vi "Multicolumn Sort.vi"(10 "Imported Details":string[][](array[string])=array424x42[17808 elements], 11 "Dataset Metadata":T2={"Dataset Name"="CryoProber_MCT_Std_Diode_Summary INNER JOIN CryoProber_MCT_Std_Sample_Summary ON (CryoProber_MCT_Std_Diode_Summary.Sample_Name = CryoProber_MCT_Std_Sample_Summary.Sample_Name \nAND CryoProber_MCT_Std_Diode_Summary.Bake = CryoProber_MCT_Std_Sample_Summary.Bake)\n", "Column Headers"=["Unique_ID", "Date-Time", "Sample_Name", "Bake", "Diode_Name", "Area_(cm2)", "Diode_Pitch_(um)", "Implant_Gap_(um)", "Implant_Type", "Temperature_(K)", "TemperatureB_(K)", "Illumination", "Curve_Shape", "|J|min", "V(Jmin)", "R(Jmin)A", "I(-100)", "R(-100)A", "I(-50)", "R(-50)A", "I(-20)", "R(-20)A", "R0A", "R(+50)A", "Ideality_Factor", "Saturation_Current_Density(A/cm2)", "Series_Resistance", "Curve_Shape_Notes", "Notes", "Sample_Name", "Last_Measured_Date-Time", "Lot_ID", "Notes", "Bake", "Mask", "LayerID", "Substrate_Polarity", "Passivant", "Wavelength_Range", "Cutoff_(um)", "Best_R0A", "Wirebond_Unique_ID", "Experiment_Name", "Designed_By", "Last_Updated", "Comments", "Condition #", "Substrate"], "Header Data types"=[enum."String", enum."Date/Time", enum."String", enum."String", enum."String", enum."Double (DBL)", enum."Double (DBL)", enum."Double (DBL)", enum."String", enum."Double (DBL)", enum."Double (DBL)", enum."String", enum."String", enum."Double (DBL)", enum."Double (DBL)", enum."Single (SGL)", enum."Double (DBL)", enum."Single (SGL)", enum."Double (DBL)", enum."Single (SGL)", enum."Double (DBL)", enum."Single (SGL)", enum."Single (SGL)", enum."Single (SGL)", enum."Double (DBL)", enum."Double (DBL)", enum."Double (DBL)", enum."String", enum."String", enum."String", enum."Date/Time", enum."String", enum."String", enum."String", enum."String", enum."String", enum."String", enum."String", enum."String", enum."Double (DBL)", enum."Double (DBL)", enum."String"]}) -> (2 "Sorted Details":string[][](array[string]))   [LabVIEW 2010]
uses:
  <vilib>/addons/database/Auxilliary.llb/DB Tools DataTypes.ctl
  <vilib>/addons/database/NI_Database_API.lvlib
panel:
  in  "Delete Entry":bool
  in  "System Cancel Button":bool
  in  "System OK Button":bool
  in  "Sort Order":i32[](listbox)=[1]
  in  "Available Columns":i32[](listbox)=[6]
  # "Drag and drop"
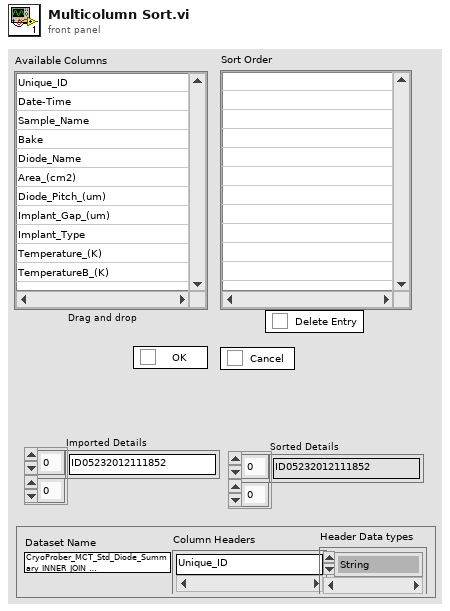
[diagram p1: front panel]
types:
  T1 = typedef "NI_Database_API.lvlib/DB Tools DataTypes.ctl" = enum16{"String", "Long (I32)", "Single (SGL)", "Double (DBL)", "Date/Time", "Binary"}
  T2 = cluster{"Dataset Name":string, "Column Headers":string[], "Header Data types":T1[]}
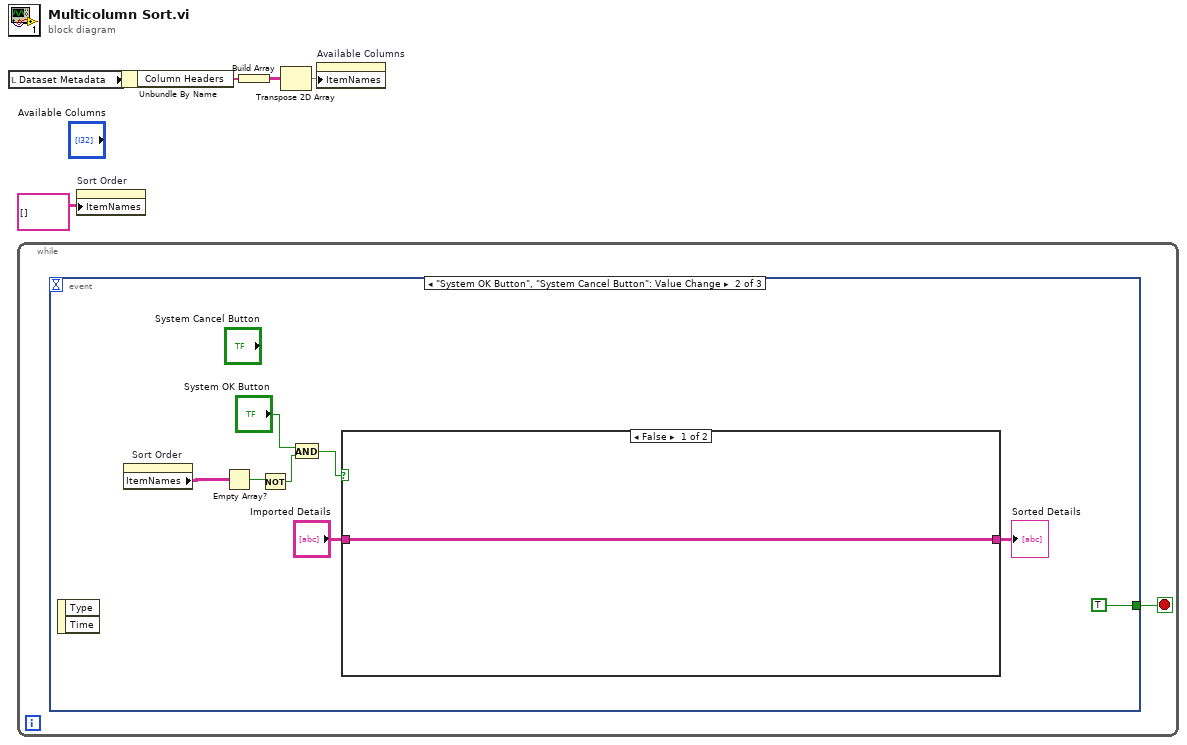
[diagram p0: block diagram]
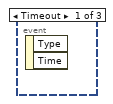
[diagram p2: hidden frame]
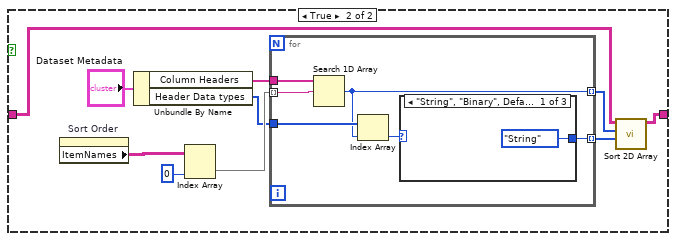
[diagram p3: hidden frame]
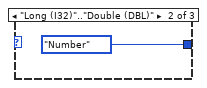
[diagram p4: hidden frame]
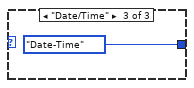
[diagram p5: hidden frame]
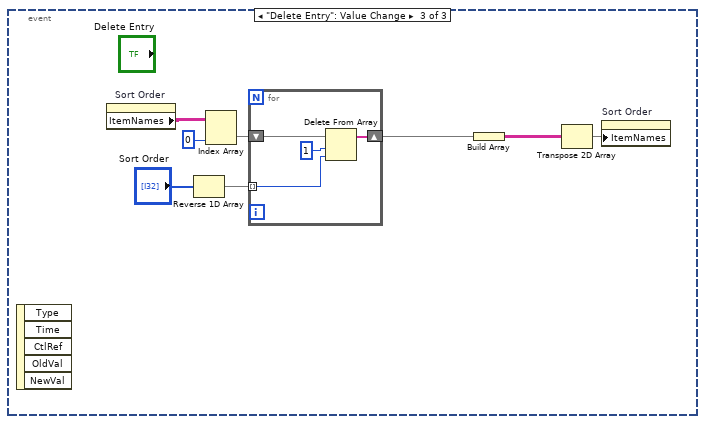
[diagram p6: hidden frame]
diagram:
  n1 = local read "Dataset Metadata"() -> (w4:T2)
  n2 = while {
    stop <- w6 stop-if-true
    n3 = event shown="[1] \"System OK Button\", \"System Cancel Button\": Value Change" {
      selector: _ -> [_ _ _]
      dyn-events: _ -> [_ _ _]
      timeout: _ -> [_ _ _]
      tunnel: [_ TRUE _] -> w6
      event Timeout {
        n4 = event-data() -> ()  [unwired: 1 in, 2 out]
      }
      event "System OK Button", "System Cancel Button": Value Change {
        n5 = event-data() -> ()  [unwired: 1 in, 2 out]
        n6 = property on="Sort Order" class="MCListbox (strict)"() -> ("ItemNames"=w13:string[][])  [unwired: 2 in, 2 out]
        n7 = Empty Array?(array=w13) -> (empty?=w10:bool)
        n8 = Not(x=w10) -> (.not. x?=w8:bool)
        n9 = And(x="System OK Button", y=w8) -> (x .and. y?=w7:bool)
        n10 = case shown="False" w7 {
          tunnel: [w15 w17] -> w12
          tunnel: "Imported Details" -> [w15 w16]
          frame False {
          }
          frame True {
            n11 = property on="Sort Order" class="MCListbox (strict)"() -> ("ItemNames"=w25:string[][])  [unwired: 2 in, 2 out]
            n12 = Unbundle By Name("Dataset Metadata") -> ("Column Headers"=w21:string[], "Header Data types"=w19:T1[])
            n13 = Index Array(array=w25, index (col)=0 ("disabled index (col)")) -> (element=w23:string[])  [unwired: 1 in]
            n14 = for {
              tunnel: w23 -> [w31] mode=indexing
              tunnel: w21 -> [w30]
              tunnel: [w28] -> w20 mode=indexing
              tunnel: w19 -> [w29]
              tunnel: [w26] -> w18 mode=indexing
              n15 = Search 1D Array(1D array=w30, element=w31) -> (index of element=w28:i32)  [unwired: 1 in]
              n16 = Index Array(array=w29, index=w28) -> (element=w27:T1)
              n17 = case shown="\"String\", \"Binary\", Default" w27 {
                tunnel: [enum16{"String", "Number", "Date-Time"}."String" ("Sort Type") enum16{"String", "Number", "Date-Time"}."Number" ("Sort Type") enum16{"String", "Number", "Date-Time"}."Date-Time" ("Sort Type")] -> w26
                frame "String", "Binary", Default {
                }
                frame "Long (I32)".."Double (DBL)" {
                }
                frame "Date/Time" {
                }
              }
            }
            n18 = call "Sort 2D Array.vi"("Sort by Datatype Array"=w18, "Sort by Cols"=w20, "Input Array"=w16) -> ("Output Array"=w17:string[][])  [unwired: 8 in]
          }
        }
        "Sorted Details" <- w12
      }
      event "Delete Entry": Value Change {
        n19 = event-data() -> ()  [unwired: 1 in, 5 out]
        n20 = property on="Sort Order" class="MCListbox (strict)"() -> ("ItemNames"=w40:string[][])  [unwired: 2 in, 2 out]
        n21 = Reverse 1D Array(array="Sort Order") -> (reversed array=w41:i32[])
        n22 = Index Array(array=w40, index (col)=0 ("disabled index (col)")) -> (element=w38:string[])  [unwired: 1 in]
        n23 = for {
          tunnel: w41 -> [w44] mode=indexing
          shift-right: [w45] -> w37
          shift-left: w38 -> [w46]
          n24 = Delete From Array(array=w46, length=1, index=w44) -> (array with subset deleted=w45:string[])  [unwired: 1 out]
        }
        n25 = Build Array(w37) -> (w36:string[][])
        n26 = Transpose 2D Array(2D array=w36) -> (transposed array=w35:string[][])
        n27 = property on="Sort Order" class="MCListbox (strict)"("ItemNames"=w35) -> ()  [unwired: 2 in, 2 out]
      }
    }
  }
  n28 = property on="Sort Order" class="MCListbox (strict)"("ItemNames"=string[][] [] ("Item Names")) -> ()  [unwired: 2 in, 2 out]
  n29 = Unbundle By Name(w4) -> ("Column Headers"=w3:string[])
  n30 = Build Array(w3) -> (w2:string[][])
  n31 = Transpose 2D Array(2D array=w2) -> (transposed array=w1:string[][])
  n32 = property on="Available Columns" class="MCListbox (strict)"("ItemNames"=w1) -> ()  [unwired: 2 in, 2 out]
